vi "sinanju_goto.vi"(3 "错误输入（无错误）":errorcluster, 4 "t":sgl, 5 "z1":sgl, 6 "y1":sgl, 7 "x1":sgl, 8 "mode":i32, 9 "page":i32, 10 "ax":i32, 11 "VISA资源名称":refnum<visa-resource-name>) -> (1 "错误输出":errorcluster, 2 "VISA资源名称输出":refnum<visa-resource-name>)   [LabVIEW 2017]
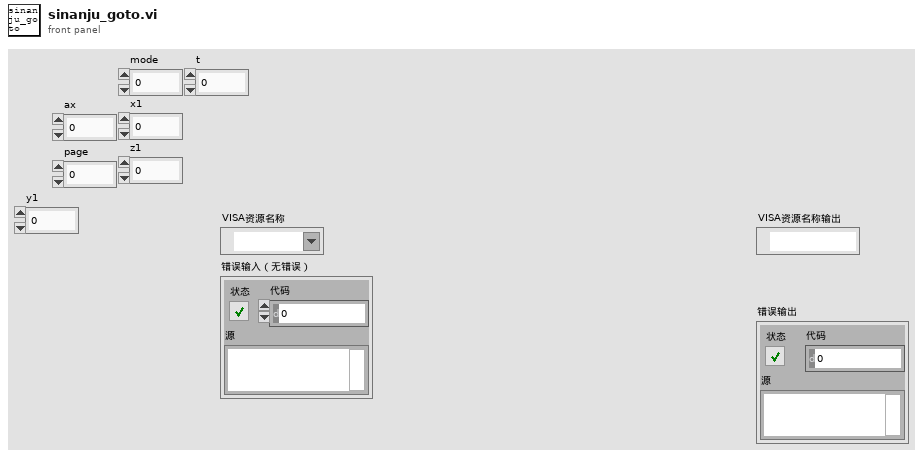
[diagram p1: front panel]
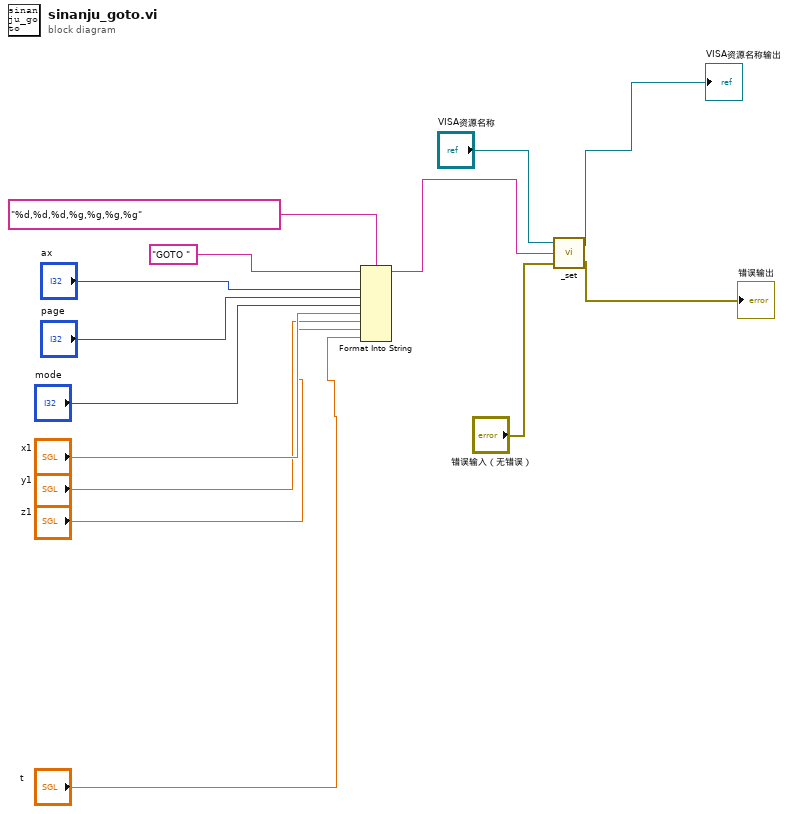
[diagram p0: block diagram]
diagram:
  n1 = Format Into String(format string="%d,%d,%d,%g,%g,%g,%g" ("格式字符串"), initial string="GOTO " ("初始字符串"), "ax", "page", "mode", "x1", "y1", "z1", "t") -> (resulting string=w9:string)  [unwired: 1 in, 1 out]
  n2 = call "_set.vi"("错误输入（无错误）"="错误输入（无错误）", "写入缓冲区"=w9, "VISA资源名称输出 2"="VISA资源名称") -> ("错误输出"=→"错误输出":errorcluster, "VISA资源名称输出"=→"VISA资源名称输出":refnum<visa-resource-name>)
